vi "Day 4 - build set.vi"(11 "String (a-b)":string) -> (3 "Set (a..b inclusive)":set{i32}(c389))   [LabVIEW 2020]
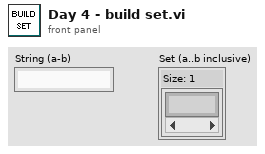
[diagram p1: front panel]
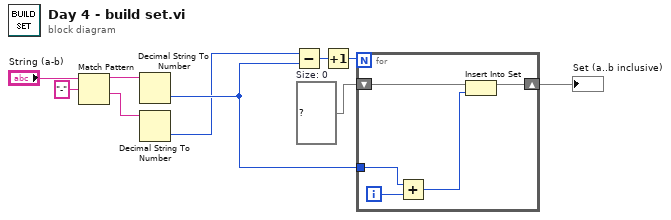
[diagram p0: block diagram]
diagram:
  w7 = set{i32} {}  # Size: 0
  n1 = Match Pattern(string="String (a-b)", regular expression="-") -> (before substring=w6:string, after substring=w5:string)  [unwired: 1 in, 2 out]
  n2 = Decimal String To Number(string=w6) -> (number=w2:i32)  [unwired: 2 in, 1 out]
  n3 = Decimal String To Number(string=w5) -> (number=w1:i32)  [unwired: 2 in, 1 out]
  n4 = Subtract(x=w1, y=w2) -> (x-y=w9:i32)
  n5 = Increment(x=w9) -> (x+1=w8:i32)
  n6 = for {
    N: w8 -> [_]
    shift-right: [w12] -> w10
    shift-left: w7 -> [w15]
    tunnel: w2 -> [w11]
    i -> [w14]
    n7 = Add(x=w11, y=w14) -> (x+y=w13:i32)
    n8 = Insert Into Set(10:w13, 11:w15) -> (3:w12:set{i32})  [unwired: 1 out]
  }
  "Set (a..b inclusive)" <- w10
